vi "Polarity_sign_array.vi"(8 "CAEN 2 in":T1, 11 "CAEN 1 in":T1) -> (0 "CAEN 2 out":T1, 2 "Polarity signs":i32[](array[numeric]), 3 "CAEN 1 out":T1)   [LabVIEW 2018]
uses:
  <instrlib>/CAEN PSM/CAEN PSM.lvlib
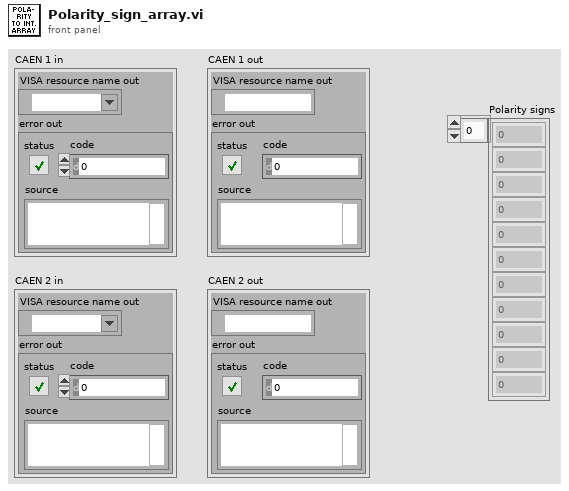
[diagram p1: front panel]
types:
  T1 = cluster{"VISA resource name out":refnum<visa-resource-name>, "error out":errorcluster}
  T2 = cluster{"VISA resource name out":refnum<visa-resource-name>, i32, i32}
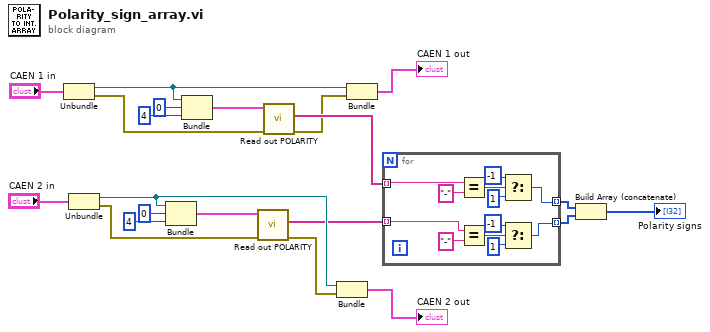
[diagram p0: block diagram]
diagram:
  n1 = Unbundle("CAEN 1 in") -> ("VISA resource name out"=w8:refnum<visa-resource-name>, "error out"=w7:errorcluster)
  n2 = Unbundle("CAEN 2 in") -> ("VISA resource name out"=w16:refnum<visa-resource-name>, "error out"=w14:errorcluster)
  n3 = Bundle("VISA resource name out"=w16, 0, 4) -> (w13:T2)  [unwired: 1 in]
  n4 = Bundle("VISA resource name out"=w8, 0, 4) -> (w6:T2)  [unwired: 1 in]
  n5 = call <instrlib>:"Read out POLARITY.vi"("error in (no error)"=w14, "BoardHandle"=w13) -> ("error out"=w17:errorcluster, "Polarity values"=w15:string[])  [unwired: 7 in, 1 out]
  n6 = call <instrlib>:"Read out POLARITY.vi"("error in (no error)"=w7, "BoardHandle"=w6) -> ("error out"=w2:errorcluster, "Polarity values"=w3:string[])  [unwired: 7 in, 1 out]
  n7 = Bundle("VISA resource name out"=w16, "error out"=w17) -> (→"CAEN 2 out":T1)  [unwired: 1 in]
  n8 = Bundle("VISA resource name out"=w8, "error out"=w2) -> (→"CAEN 1 out":T1)  [unwired: 1 in]
  n9 = for {
    tunnel: w3 -> [w33] mode=indexing
    tunnel: [w28] -> w19 mode=indexing
    tunnel: w15 -> [w23] mode=indexing
    tunnel: [w22] -> w20 mode=indexing
    n10 = Equal?(x=w33, y="-") -> (x = y?=w31:bool)
    n11 = Equal?(x=w23, y="-") -> (x = y?=w26:bool)
    n12 = Select(t=-1, s=w31, f=1) -> (s? t:f=w28:i32)
    n13 = Select(t=-1, s=w26, f=1) -> (s? t:f=w22:i32)
  }
  n14 = Build Array (concatenate)(w19, w20) -> (→"Polarity signs":i32[])
